vi "Grab and save data for ace_v2.vi"() -> ()   [LabVIEW 2014]
doc: "This VI is used to acquire image into computer memory for further processing, e.g. real-time height feedback by analyzing stuck bead ring pattern, or saving images while doing force clamp feedback.\nThis VI grabs image from CCD and extracts single stuck bead image to a global variable.Remember not to turn off this VI since all image sourses from here, while other VIs are acquiring images. \nIn LabVIEW, input image data is saved into memory and is assigned a memory address. The image control or indicator only passes the memory address not whole image data. Thus, one should create lots of memory addresses, or new input image will overwrite the previous one. In the case of running force clamp and image synchronization VI, and due to the limitation of CCD rate, this VI usually creates 80 memory addresses for image temporarily saving, which can save continuous 2 seconds image waiting for saving.\n\nThis VI is designed based on NI vi example\"Grab.vi\", thus in a high-speed capture mode. (Snap.vi is a low-speed capture mode).\n\nThe Grab VI acquires images continuously and displays the images in an image control using high-level acquisition VIs. A grab is appropriate for high-speed applications in which you need to process only one image at a time.\n\nThe Snap VI acquires an image and displays the image in an image control using low-level acquisition VIs. A snap is appropriate for low-speed or single-capture applications in which ease of programming is essential."
uses:
  <vilib>/userdefined/High Color/IMAQdx.ctl
  <vilib>/vision/Image Controls.llb/IMAQ Image.ctl
  Global 1 extract image.vi
  <vilib>/vision/driver/NI_Vision_Acquisition_Software.lvlib
  <vilib>/vision/NI_Vision_Development_Module.lvlib
panel:
  out "error out":errorcluster
  in  "Extract ot not":bool
  in  "# Of Buffers":i32=80
  out "Time (s)":dbl
  out "Buffer Number Out":u32
  in  "Turn OFF camera?":bool
  in  "take pic?":bool=TRUE
  out "Y Resolution of Extract":i32
  out "X Resolution of Extract":i32
  out "Image with Extract":T1(plugin-control)
  in  "Stop Grab Image":bool
  in  "Camera Name":T2="cam1"
  out "Original Image":T1(plugin-control)
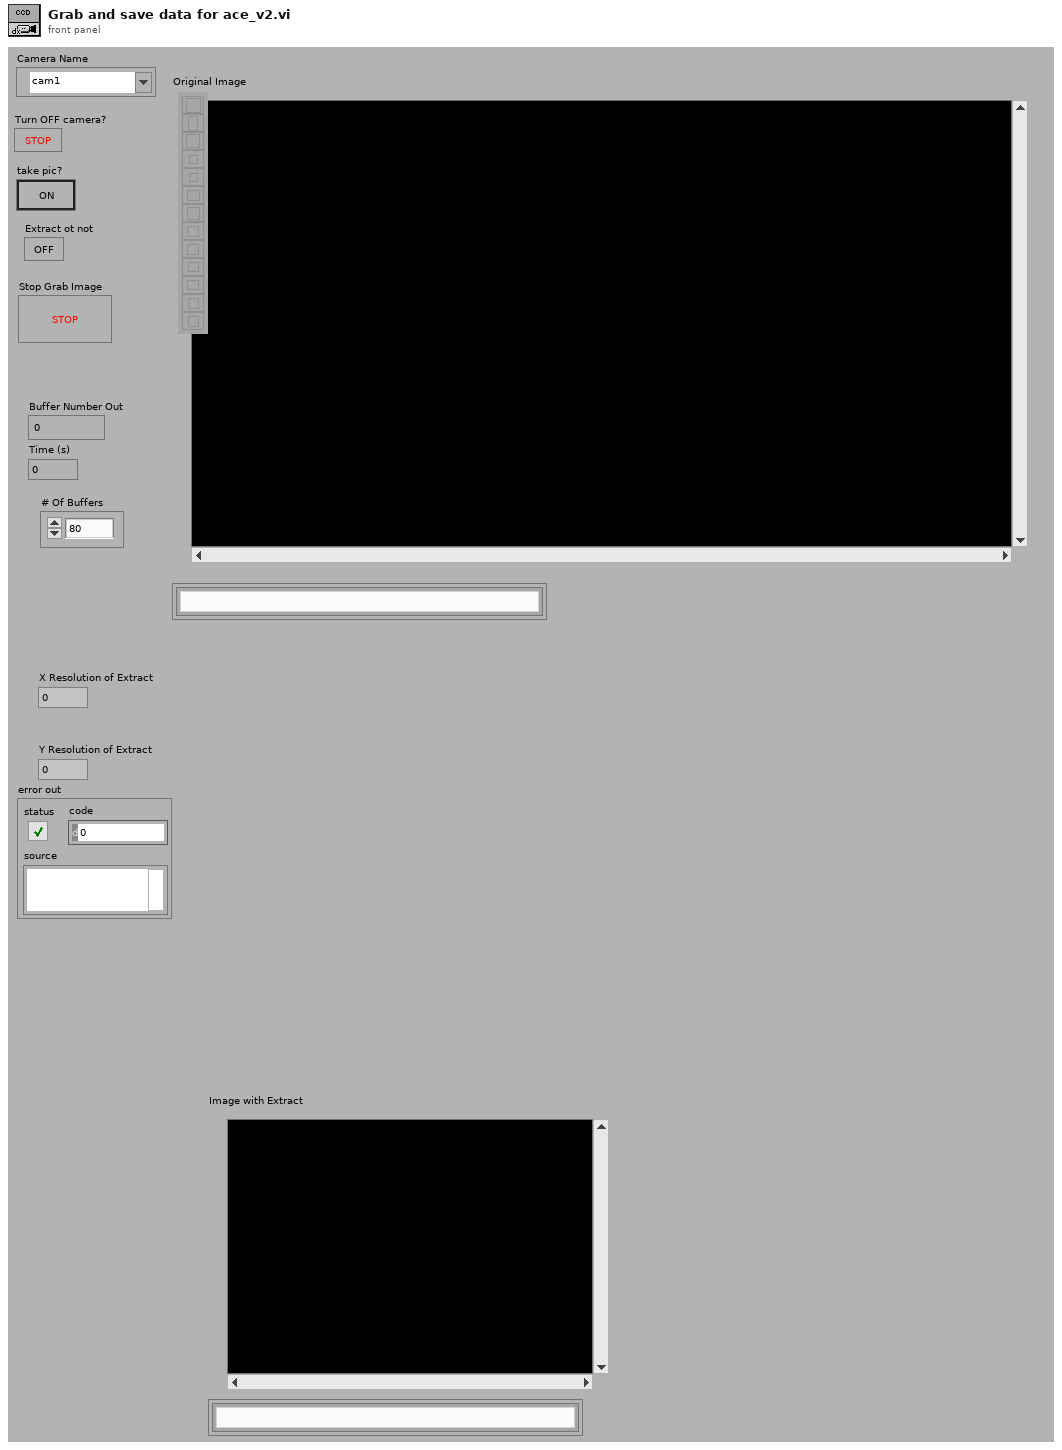
[diagram p1: front panel]
types:
  T1 = typedef "IMAQ Image.ctl" = refnum<image>
  T2 = typedef "IMAQdx.ctl" = refnum<k21>
  T3 = typedef "Image Type" = u32
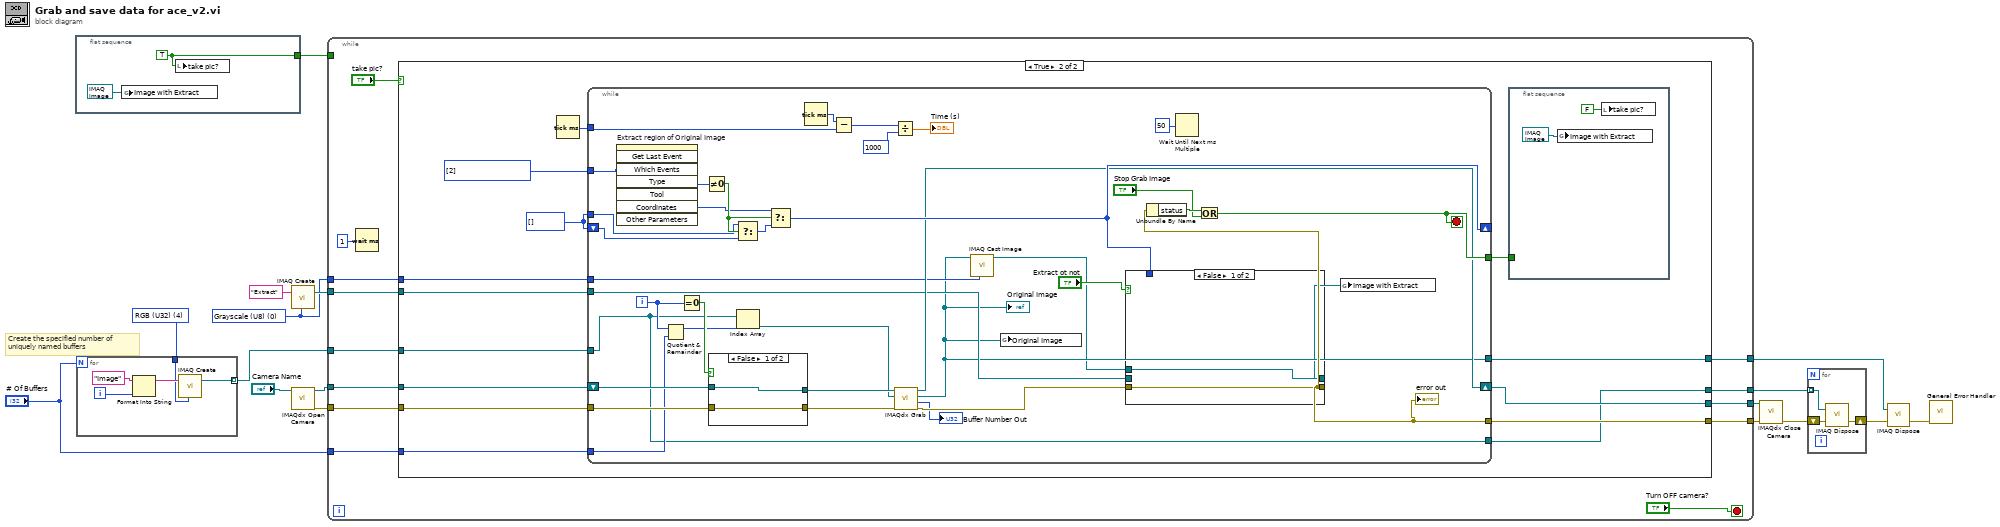
[diagram p0: block diagram]
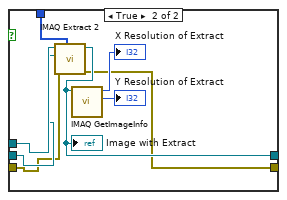
[diagram p3: hidden frame]
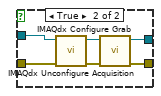
[diagram p4: hidden frame]
diagram:
  w1 = T3 0 items=["Grayscale (U8)", "Grayscale (I16)", "Grayscale (SGL)", "Complex (CSG)", "RGB (U32)", "HSL (U32)", "RGB (U64)", "Grayscale (U16)"] ("Image Type")
  w5 = T3 4 items=["Grayscale (U8)", "Grayscale (I16)", "Grayscale (SGL)", "Complex (CSG)", "RGB (U32)", "HSL (U32)", "RGB (U64)", "Grayscale (U16)"] ("Image Type")
  # "Create the specified number of \nuniquely named buffers"
  n1 = flat-sequence {
    tunnel: [w18] -> w7
    frame #0 {
      w18 = TRUE
      n2 = global write "Global 1 extract image.vi" "Image with Extract"(T1 refnum ("Image with Extract")) -> ()
      n3 = local write "take pic?"(w18) -> ()
    }
  }
  n4 = for {
    N: "# Of Buffers" -> [_]
    tunnel: [w24] -> w4 mode=indexing
    tunnel: w5 -> [w20]
    i -> [w23]
    n5 = Format Into String(initial string="Image" ("Image Name"), w23) -> (resulting string=w21:string)  [unwired: 2 in, 1 out]
    n6 = call "IMAQ Create"("Image Name"=w21, "Image Type"=w20) -> ("New Image"=w24:T1)  [unwired: 3 in, 1 out]
  }
  n7 = call "IMAQ Create"("Image Name"="Extract", "Image Type"=w1) -> ("New Image"=w8:T1)  [unwired: 2 in, 2 out]
  n8 = call <vilib>:"IMAQdx Open Camera.vi"("Session In"="Camera Name") -> ("error out"=w9:errorcluster, "Session Out"=w10:T2)  [unwired: 2 in, 7 out]
  n9 = while {
    tunnel: [w37] -> w15
    tunnel: [w36] -> w14
    tunnel: [w35] -> w13
    tunnel: w10 -> [w34]
    tunnel: w9 -> [w33]
    tunnel: w4 -> [w32]
    tunnel: w8 -> [w31]
    tunnel: w7 -> [_]
    tunnel: "# Of Buffers" -> [w27]
    tunnel: [w26] -> w3
    tunnel: w1 -> [w25]
    stop <- "Turn OFF camera?" stop-if-true
    n10 = Wait (ms)(milliseconds to wait=u32 1) -> ()  [unwired: 1 out]
    n11 = case shown="True" "take pic?" {
      tunnel: [w39 w43] -> w26
      tunnel: [w40 w54] -> w37
      tunnel: [w41 w53] -> w36
      tunnel: [w38 w52] -> w35
      tunnel: w34 -> [w41 w51]
      tunnel: w33 -> [w40 w50]
      tunnel: w32 -> [w39 w49]
      tunnel: w31 -> [w38 w48]
      tunnel: w27 -> [_ w44]
      tunnel: w25 -> [_ w42]
      frame False {
      }
      frame True {
        w55 = i32[] [2] items=["No  event", "Click event", "Draw event", "Move event", "Size event", "Scroll event", "Activate event", "Close event", "Double click event"] ("Events list (all)")
        w45 = i32[] [] ("Coordinates")
        n12 = Tick Count (ms)() -> (millisecond timer value=w46:u32)
        n13 = while {
          tunnel: [w62] -> w54
          tunnel: w50 -> [w84]
          tunnel: [w60] -> w52
          shift-right: [w83] -> _
          shift-left: w45 -> [w87]
          tunnel: w55 -> [w92]
          tunnel: w45 -> [w86]
          shift-right: [w74] -> w53
          shift-left: w51 -> [w85]
          tunnel: w49 -> [w65]
          tunnel: w48 -> [w63]
          tunnel: [w81] -> w47
          tunnel: w46 -> [w79]
          tunnel: w44 -> [w68]
          tunnel: [w65] -> w43
          tunnel: w42 -> [w61]
          i -> [w69]
          stop <- w81 stop-if-true
          n14 = invoke on="Extract region of Original Image" class="ImageControl" method="Get Last Event"("Which Events"=w92) -> ("Type"=w91:i32, "Coordinates"=w88:i32[])  [unwired: 7 in, 6 out]
          n15 = Quotient & Remainder(x=w69, y=w68) -> (x-y*floor(x/y)=w67:i32)  [unwired: 1 out]
          n16 = Equal To 0?(x=w69) -> (x = 0?=w82:bool)
          n17 = Not Equal To 0?(x=w91) -> (x != 0?=w90:bool)
          n18 = case shown="False" w82 {
            tunnel: w85 -> [w106 w112]
            tunnel: w84 -> [w105 w111]
            tunnel: [w106 w110] -> w75
            tunnel: [w105 w109] -> w73
            frame False {
            }
            frame True {
              n19 = call <vilib>:"IMAQdx Unconfigure Acquisition.vi"("error in"=w111, "Session In"=w112) -> ("error out"=w107:errorcluster, "Session Out"=w108:T2)  [unwired: 8 out]
              n20 = call <vilib>:"IMAQdx Configure Grab.vi"("error in"=w107, "Session In"=w108) -> ("error out"=w109:errorcluster, "Session Out"=w110:T2)  [unwired: 1 in, 7 out]
            }
          }
          n21 = Select(t=w86, s=w90, f=w87) -> (s? t:f=w89:i32[])
          n22 = Index Array(array=w65, index=w67) -> (element=w66:T1)
          n23 = Select(t=w88, s=w90, f=w89) -> (s? t:f=w83:i32[])
          n24 = Tick Count (ms)() -> (millisecond timer value=w80:u32)
          n25 = Subtract(x=w80, y=w79) -> (x-y=w78:u32)
          n26 = Divide(x=w78, y=u32 1000) -> (x/y=→"Time (s)":dbl)
          n27 = call <vilib>:"IMAQdx Grab.vi"("error in"=w73, "Image In"=w66, "Session In"=w75) -> ("error out"=w72:errorcluster, "Buffer Number Out"=→"Buffer Number Out":u32, "Image Out"=w60:T1, "Session Out"=w74:T2)  [unwired: 5 in]
          "Original Image" <- w60
          n28 = call "IMAQ Cast Image"("Image Type"=w61, "Image Src"=w60) -> ("Image Dst Out"=w59:T1)  [unwired: 8 in, 1 out]
          n29 = global write "Global 1 extract image.vi" "Original Image"(w60) -> ()
          n30 = case shown="False" "Extract ot not" {
            tunnel: w83 -> [_ w102]
            tunnel: [w95 w100] -> w62
            tunnel: w59 -> [w96 w99]
            tunnel: w72 -> [w95 w97]
            tunnel: [w96 w101] -> w58
            tunnel: w63 -> [_ w98]
            frame False {
            }
            frame True {
              n31 = call "IMAQ Extract 2"("Optional Rectangle"=w102, "error in (no error)"=w97, "Image Dst"=w98, "Image Src"=w99) -> ("error out"=w100:errorcluster, "Image Dst Out"=w101:T1)  [unwired: 6 in]
              "Image with Extract" <- w101
              n32 = call "IMAQ GetImageInfo"("Image"=w101) -> ("Y Resolution"=→"Y Resolution of Extract":i32, "X Resolution"=→"X Resolution of Extract":i32)  [unwired: 1 in, 8 out]
            }
          }
          "error out" <- w62
          n33 = Unbundle By Name(w62) -> ("status"=w94:bool)
          n34 = Wait Until Next ms Multiple(millisecond multiple=u32 50) -> ()  [unwired: 1 out]
          n35 = Or(x=w94, y="Stop Grab Image") -> (x .or. y?=w81:bool)
          n36 = global write "Global 1 extract image.vi" "Image with Extract"(w58) -> ()
        }
        n37 = flat-sequence {
          tunnel: w47 -> [_]
          frame #0 {
            n38 = global write "Global 1 extract image.vi" "Image with Extract"(T1 refnum ("Image with Extract")) -> ()
            n39 = local write "take pic?"(FALSE) -> ()
          }
        }
      }
    }
  }
  n40 = call <vilib>:"IMAQdx Close Camera.vi"("error in"=w15, "Session In"=w14) -> ("error out"=w16:errorcluster)  [unwired: 9 out]
  n41 = for {
    shift-right: [w115] -> w17
    shift-left: w16 -> [w114]
    tunnel: w3 -> [w113] mode=indexing
    n42 = call "IMAQ Dispose"("Image"=w113, "error in (no error)"=w114) -> ("error out"=w115:errorcluster)  [unwired: 1 in, 3 out]
  }
  n43 = call "IMAQ Dispose"("Image"=w13, "error in (no error)"=w17) -> ("error out"=w2:errorcluster)  [unwired: 1 in, 3 out]
  n44 = call <vilib>:"General Error Handler.vi"("error in (no error)"=w2) -> ()  [unwired: 2 in, 13 out]
